vi "WireCallParent.vi"(2 "error in (no error)":errorcluster, 3 "classesVIPath":path) -> (0 "error out":errorcluster)   [LabVIEW 2009, in "HGF_VisitorGenerator.lvlib"]
doc: "wire call parent VI inputs (action.vi)"
uses:
  HGF_VisitorGenerator.lvlib
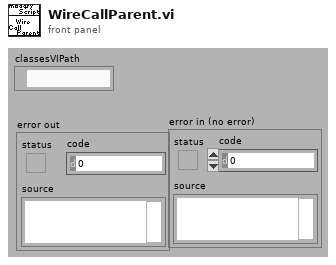
[diagram p1: front panel]
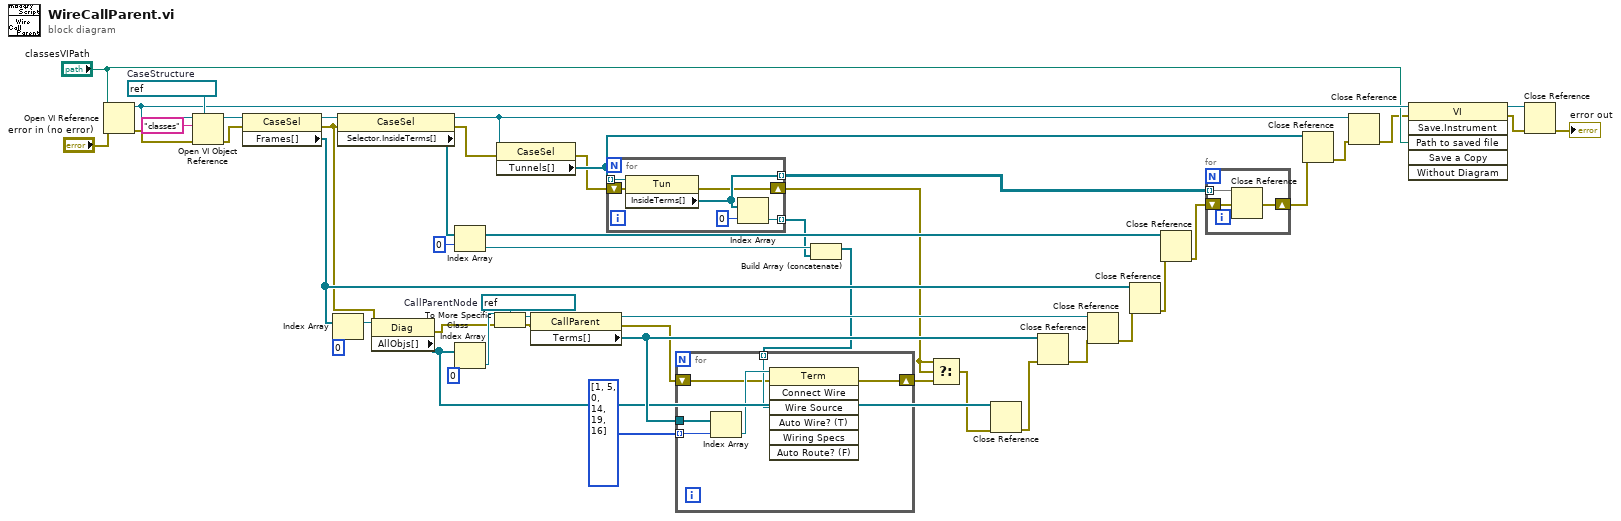
[diagram p0: block diagram]
diagram:
  w32 = refnum<vi> refnum  # CaseStructure
  w39 = refnum<vi> refnum  # CallParentNode
  n1 = Open VI Reference(vi path="classesVIPath", error in (no error)="error in (no error)") -> (vi reference=w27:refnum<vi>, error out=w30:errorcluster)  [unwired: 4 in]
  n2 = Open VI Object Reference(7:w32, 8:w30, 10:"classes" ("name/order"), 11:w27) -> (0:w29:errorcluster, 3:w33:refnum<vi>)
  n3 = property class="CaseSel"(reference=w33, error in=w29) -> (reference out=w47:refnum<vi>, error out=w42:errorcluster, "Frames[]"=w45:refnum<vi>[])
  n4 = Index Array(array=w45, index=0) -> (element=w14:refnum<vi>)
  n5 = property class="CaseSel"(reference=w47, error in=w42) -> (reference out=w13:refnum<vi>, error out=w5:errorcluster, "Selector.InsideTerms[]"=w23:refnum<vi>[])
  n6 = property class="Diag"(reference=w14, error in=w42) -> (error out=w37:errorcluster, "AllObjs[]"=w7:refnum<vi>[])  [unwired: 1 out]
  n7 = Index Array(array=w23, index=0) -> (element=w17:refnum<vi>)
  n8 = Index Array(array=w7, index=0) -> (element=w38:refnum<vi>)
  n9 = To More Specific Class(target class=w39, reference=w38, error in=w37) -> (specific class reference=w40:refnum<vi>, error out=w41:errorcluster)
  n10 = property class="CaseSel"(reference=w13, error in=w5) -> (error out=w4:errorcluster, "Tunnels[]"=w12:refnum<vi>[])  [unwired: 1 out]
  n11 = property class="CallParent"(reference=w40, error in=w41) -> (reference out=w36:refnum<vi>, error out=w15:errorcluster, "Terms[]"=w21:refnum<vi>[])
  n12 = for {
    tunnel: w12 -> [w54] mode=indexing
    tunnel: [w52] -> w11 mode=indexing
    tunnel: [w51] -> w10 mode=indexing
    shift-right: [w49] -> w2
    shift-left: w4 -> [w50]
    n13 = property class="Tun"(reference=w54, error in=w50) -> (error out=w49:errorcluster, "InsideTerms[]"=w51:refnum<vi>[])  [unwired: 1 out]
    n14 = Index Array(array=w51, index=0) -> (element=w52:refnum<vi>)
  }
  n15 = Build Array (concatenate)(w17, w11) -> (w16:refnum<vi>[])
  n16 = for {
    tunnel: w21 -> [w60]
    shift-right: [w59] -> w3
    shift-left: w15 -> [w55]
    tunnel: i32[] [1, 5, 0, 14, 19, 16] -> [w57] mode=indexing
    tunnel: w16 -> [w56] mode=indexing
    n17 = Index Array(array=w60, index=w57) -> (element=w58:refnum<vi>)
    n18 = invoke class="Term" method="Connect Wire"(reference=w58, error in=w55, "Wire Source"=w56) -> (error out=w59:errorcluster)  [unwired: 4 in, 6 out]
  }
  n19 = Select(t=w2, s=w2, f=w3) -> (s? t:f=w1:errorcluster)
  n20 = Close Reference(reference=w7, error in (no error)=w1) -> (error out=w6:errorcluster)
  n21 = Close Reference(reference=w21, error in (no error)=w6) -> (error out=w35:errorcluster)
  n22 = Close Reference(reference=w36, error in (no error)=w35) -> (error out=w46:errorcluster)
  n23 = Close Reference(reference=w45, error in (no error)=w46) -> (error out=w48:errorcluster)
  n24 = Close Reference(reference=w23, error in (no error)=w48) -> (error out=w9:errorcluster)
  n25 = for {
    tunnel: w10 -> [w63] mode=indexing
    shift-right: [w61] -> w8
    shift-left: w9 -> [w62]
    n26 = Close Reference(reference=w63, error in (no error)=w62) -> (error out=w61:errorcluster)
  }
  n27 = Close Reference(reference=w12, error in (no error)=w8) -> (error out=w18:errorcluster)
  n28 = Close Reference(reference=w13, error in (no error)=w18) -> (error out=w19:errorcluster)
  n29 = invoke class="VI" method="Save.Instrument"(reference=w27, error in=w19, "Path to saved file"="classesVIPath") -> (reference out=w26:refnum<vi>, error out=w25:errorcluster)  [unwired: 3 in, 4 out]
  n30 = Close Reference(reference=w26, error in (no error)=w25) -> (error out=→"error out":errorcluster)
